vi "Config - Update.vi"(8 "error in (no error)":errorcluster, 10 "Config Data":T2 {"Balance" format="%9.2g"}, 11 "Config Array":T1 {"Balance" format="%9.2g"}) -> (0 "error out":errorcluster, 3 "Config Array":T1 {"Balance" format="%9.2g"})   [LabVIEW 2017]
doc: "Provides Update mechanism in Config Array by Config Data portion."
uses:
  Controls/Config Array.ctl
  Controls/Config Data.ctl
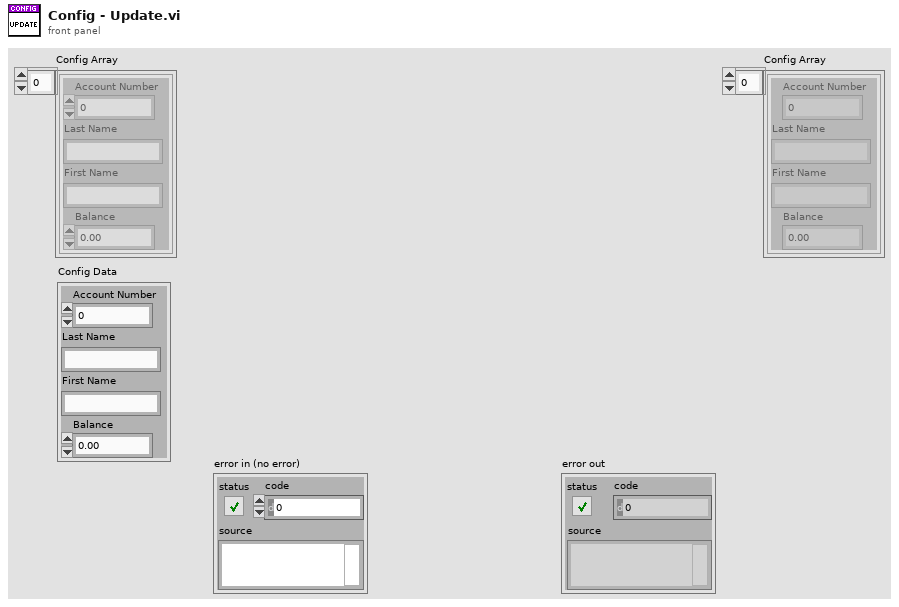
[diagram p1: front panel]
types:
  T1 = typedef "Config Array.ctl" = T2[]
  T2 = typedef "Config Data.ctl" = cluster{"Account Number":u32, "Last Name":string, "First Name":string, "Balance":dbl}
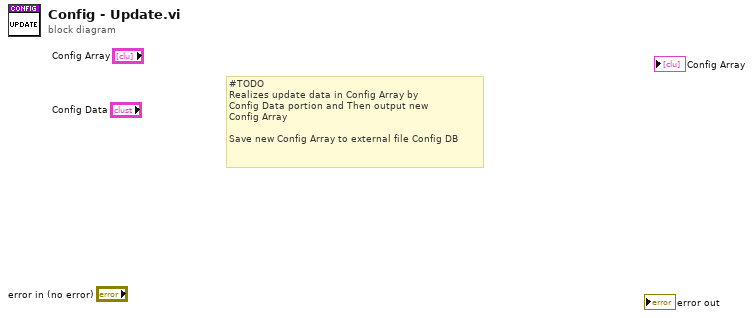
[diagram p0: block diagram]
diagram:
  # "#TODO\nRealizes update data in Config Array by\nConfig Data portion and Then output new\nConfig Array\n\nSave new Config Array to external file Config DB"
